vi "output.vi"(8 "error in (no error)":errorcluster caption="错误输入（无错误）", 11 "ShopBase输入":refnum<class "ShopBase.lvclass">) -> (0 "error out":errorcluster caption="错误输出", 2 "布尔":bool, 3 "ShopBase输出":refnum<class "ShopBase.lvclass">)   [LabVIEW 2013, in "ShopBase.lvclass"]
uses:
  ShopBase.lvclass
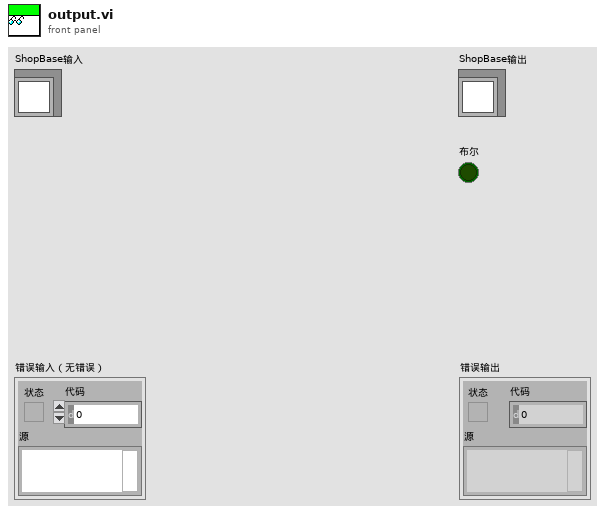
[diagram p1: front panel]
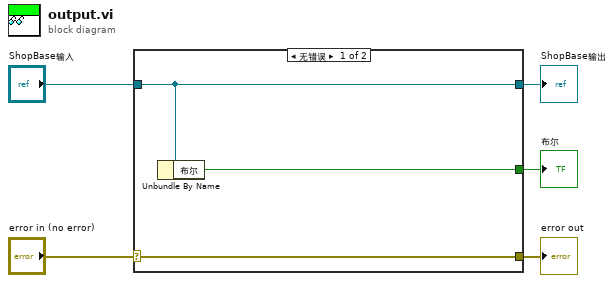
[diagram p0: block diagram]
diagram:
  n1 = case shown="无错误" "error in (no error)" {
    selector: "error in (no error)" -> [w8 w9]
    tunnel: [w8 w9] -> w4
    tunnel: [w7 w10] -> w2
    tunnel: "ShopBase输入" -> [w7 w10]
    tunnel: [w6 _] -> w1
    frame No Error {
      n2 = Unbundle By Name(w7) -> ("布尔"=w6:bool)
    }
    frame Error {
    }
  }
  "error out" <- w4
  "ShopBase输出" <- w2
  "布尔" <- w1
